vi "Open My Data HDF5.vi"(5 "Comment":string, 7 "Time Stamp":timestamp, 8 "error in":errorcluster, 10 "Dataset Path":string, 11 "file path":path) -> (0 "error out":errorcluster, 3 "Refs":T1)   [LabVIEW 2014]
uses:
  My Data HDF5 Refs.ctl
  <vilib>/UPVI/lvhdf5/library.llb/HDF5 Ref.ctl
  <vilib>/UPVI/lvhdf5/file.llb/LVH5F Operation.ctl
  <vilib>/UPVI/lvhdf5/dataset.llb/LVH5D Operation.ctl
  <vilib>/UPVI/lvhdf5/attribute.llb/LVH5A Operation.ctl
  <vilib>/UPVI/lvhdf5/dataset.llb/Simple OpenCreateReplace Dataset (Variant).vi
  <vilib>/UPVI/lvhdf5/attribute.llb/Simple H5Awrite (Variant).vi
  <vilib>/UPVI/lvhdf5/dataset.llb/Simple OpenCreateReplace Dataset.xnode
  <vilib>/UPVI/lvhdf5/attribute.llb/Simple H5Awrite.xnode
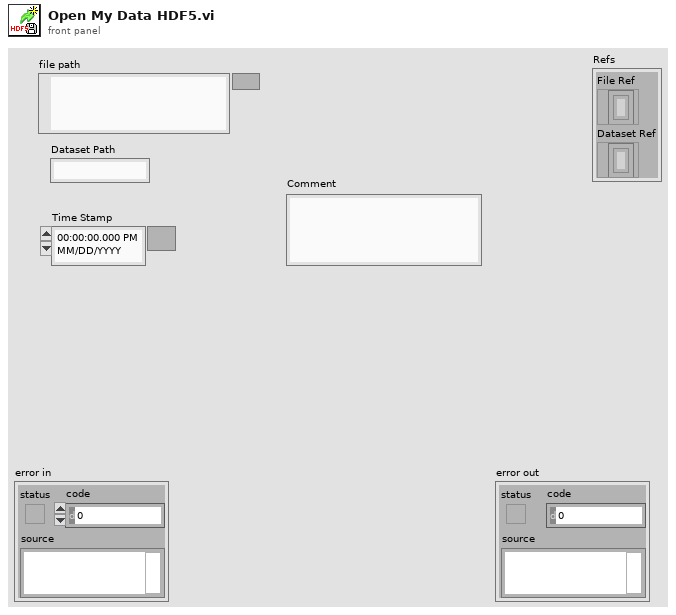
[diagram p1: front panel]
types:
  T1 = typedef "My Data HDF5 Refs.ctl" = cluster{"File Ref":T2, "Dataset Ref":T2}
  T2 = typedef "HDF5 Ref.ctl" = refnum<k1>
  T3 = cluster{"Time (s)":dbl, "Temperature (C)":dbl, "Voltage (V)":dbl}
  T4 = typedef "LVH5D Operation.ctl" = enum16{"open", "replace", "create", "open or create", "create or replace", "create or replace with confirmation"}
  T5 = typedef "LVH5F Operation.ctl" = enum16{"open", "open or create", "create or replace", "create or replace (with confirmation)", "create", "open (read only)"}
  T6 = typedef "LVH5A Operation.ctl" = enum16{"open", "replace", "create", "open or create", "create or replace", "create or replace with confirmation"}
  T7 = cluster{"Time (s)":dbl, "Temperature (C)":dbl, "Voltage (V)":dbl}[]
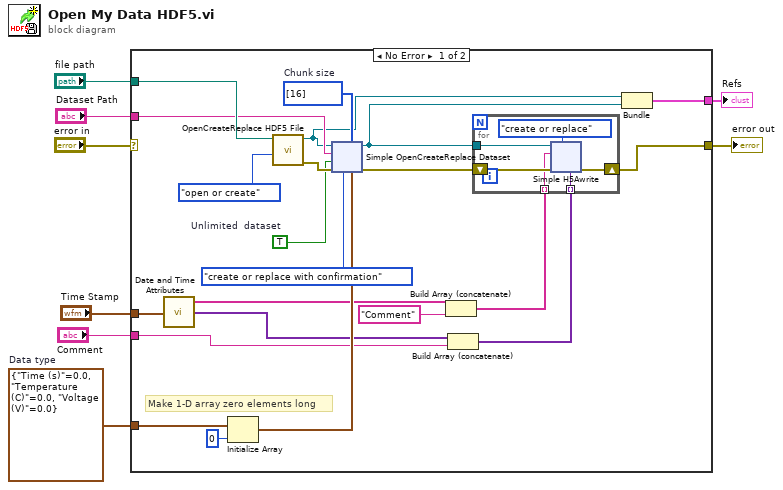
[diagram p0: block diagram]
diagram:
  w2 = T3 {"Time (s)"=0.0, "Temperature (C)"=0.0, "Voltage (V)"=0.0}  # Data type
  n1 = case shown="No Error" "error in" {
    selector: "error in" -> [_ w63]
    tunnel: [w11 w63] -> w8
    tunnel: "file path" -> [w29 _]
    tunnel: "Time Stamp" -> [w18 _]
    tunnel: "Comment" -> [w14 _]
    tunnel: "Dataset Path" -> [w28 _]
    tunnel: w2 -> [w25 _]
    tunnel: [w19 _] -> w1
    frame No Error {
      w21 = i32[] [16]  # Chunk size
      w22 = TRUE  # Unlimited  dataset
      # "Make 1-D array zero elements long"
      n2 = call <vilib>:"Date and Time Attributes.vi"("Timestamp (current)"=w18) -> ("Attribute Names"=w17:string[], "Attribute Values"=w15:variant[])  [unwired: 1 out]
      n3 = Initialize Array(w25, 0 ("dimension size")) -> (w23:T7)
      n4 = call <vilib>:"OpenCreateReplace HDF5 File.vi"("function (open or create)"=LVH5F_Operation."open or create", "path"=w29) -> ("error out"=w30:errorcluster, "HDF5 Ref out"=w20:T2)  [unwired: 6 in]
      n5 = xnode "Simple OpenCreateReplace Dataset"("Chunk size"=w21, "Dataset Path"=w28, "HDF5 Ref"=w20, "Unlimited  dataset (F)"=w22, "error in (no error)"=w30, "operation"=LVH5D_Operation."create or replace with confirmation", "Datatype and Dataspace"=w23) -> ("HDF5 Ref out"=w13:T2, "error out"=w12:errorcluster)  [unwired: 1 in, 1 out]
      n6 = Build Array (concatenate)(w17, "Comment") -> (w10:string[])
      n7 = Build Array (concatenate)(w15, w14) -> (w9:variant[])
      n8 = for {
        tunnel: w13 -> [w36]
        shift-right: [w34] -> w11
        shift-left: w12 -> [w35]
        tunnel: w10 -> [w33] mode=indexing
        tunnel: w9 -> [w32] mode=indexing
        n9 = xnode "Simple H5Awrite"("HDF5 Ref"=w36, "Name"=w33, "error in (no error)"=w35, "operation (open or create)"=LVH5A_Operation."create or replace", "Value"=w32) -> ("error out"=w34:errorcluster)  [unwired: 1 out]
      }
      n10 = Bundle("HDF5 Ref out"=w20, "HDF5 Ref out"=w13) -> (w19:cluster{"HDF5 Ref out":T2, "HDF5 Ref out":T2})  [unwired: 1 in]
    }
    frame Error {
      # "Wire previous error through"
    }
  }
  "error out" <- w8
  "Refs" <- w1
